vi "Sequencer.201806.vi"() -> ()   [LabVIEW 2014]
uses:
  Wave.ctl
  <vilib>/Analysis/NI_AALPro.lvlib
  <vilib>/gmath/NI_Gmath.lvlib
  <vilib>/gmath/statdist.llb/Poisson Random.vi
panel:
  out "Wave":T1 {"Phase (Pi)" min=-1.0 max=1.0 step=0.1 format="%.2f"; "Gap (us)" format="%.2f"; "Amplitude" format="%.2f"; "Duration (us)" format="%.2f"; "Frequency (MHz)" format="%.4f"}
  out "All Wave":T1 {"Phase (Pi)" min=-1.0 max=1.0 step=0.1 format="%.2f"; "Gap (us)" format="%.2f"; "Amplitude" format="%.2f"; "Duration (us)" format="%.2f"; "Frequency (MHz)" format="%.4f"}
  out "SegmentPositions":u32[](array[numeric])
  in  "All Wave (MHz, us, Pi)":string[][](table)=[["Frequency (MHz)", "Duration (us)", "Amplitude", "Phase (Pi)", "Gap (us)"], ["200.012", "100.000", "1.000", "0.000", "0.001"]]
  out "Item Function":refnum<vi>
  in  "Set":bool
  in  "Item":string(combo)="Time"
  out "SequenceNames":string[](array[string])
  in  "Parameter":u16(ring) items=["Frequency", "Amplitude", "Phase"]
  in  "Scan":bool
  out "Value":dbl=1.0 format="%.4f"
  in  "Step":dbl=1.0 format="%.4f"
  in  "End":dbl=1.0 format="%.3f"
  in  "Start":dbl=1.0 format="%.3f"
  out "Counts":u32[](array[numeric])
  out "CompiledSequence":string="#DopplerCooling\r\n0.9 10100000 00000000 00000000\r\n\r\n#Pump\r\n0.3 01000000 00000000 00000000\r\n\r\n#Pulsed\r\n0.2 00100000 00000000 00000000\r\n0.4 00000100 00000000 00000000\r\n0.2 00000000 10000000 00000000\r\n0.2 01000000 00000000 01000000\n"
  out "ChapterNames":string[](array[string])
  out "ChapterPositions":u32[](array[numeric])
  out "Durations Backup":dbl[](array[numeric])
  out "Durations":dbl[](array[numeric])
  in  "Period (ns)":dbl=5.0
  out "States":string[](array[string])
  in  "Sequencer":bool
  in  "Edit":enum32{"Sequence", "Wave"}(tab)
  in  "Sequence":string
  in  "Chapter (us)":string
  in  "Sequence File":path=path "D:/Data/Sequence/Cooling.seq"
  in  "Repeats":u32=100
  in  "Compile":bool
  in  "Send":bool
  in  "Port":refnum<visa-resource-name>="COM5"
  in  "Trigger":bool
  in  "Save":bool
  in  "Wave (MHz, us, Pi)":string[][](table)
  in  "Wave File":path=path "D:/Data/Wave/Test.csv"
  in  "Save":bool
  in  "Load":bool
  in  "Segment":u16(ring) items=["0"]
  in  "Index":u16(ring) items=["0", "1", "All"]
  in  "Channel":u16(ring) items=["0"]
  in  "Mode":u16(ring) items=["0"]
  out "Clock":string
  in  "Detect":enum32{"PMT", "AWG", "CCD"}(tab)
  in  "4":bool
  in  "3":bool
  in  "2":bool
  in  "1":bool=TRUE
  in  "Count or State":i16(ring) items=["Count", "State"]
  in  "Fit":bool
  out "Peak":u32
  out "?":cluster{"Axis":dbl[], "Histogram":i32[]}(graph)
  in  "Data Chapter":i16(ring) items=["All", "Detection[2]"]
  out "Average Counts or States":dbl(graph)
  out "data file":string
  out "History":dbl[](array[numeric])
  in  "Sweep":bool
  in  "Clear":bool
  in  "Data":bool
  in  "Threshold":dbl=1.0
  out "Graph":waveform(dbl)(graph)
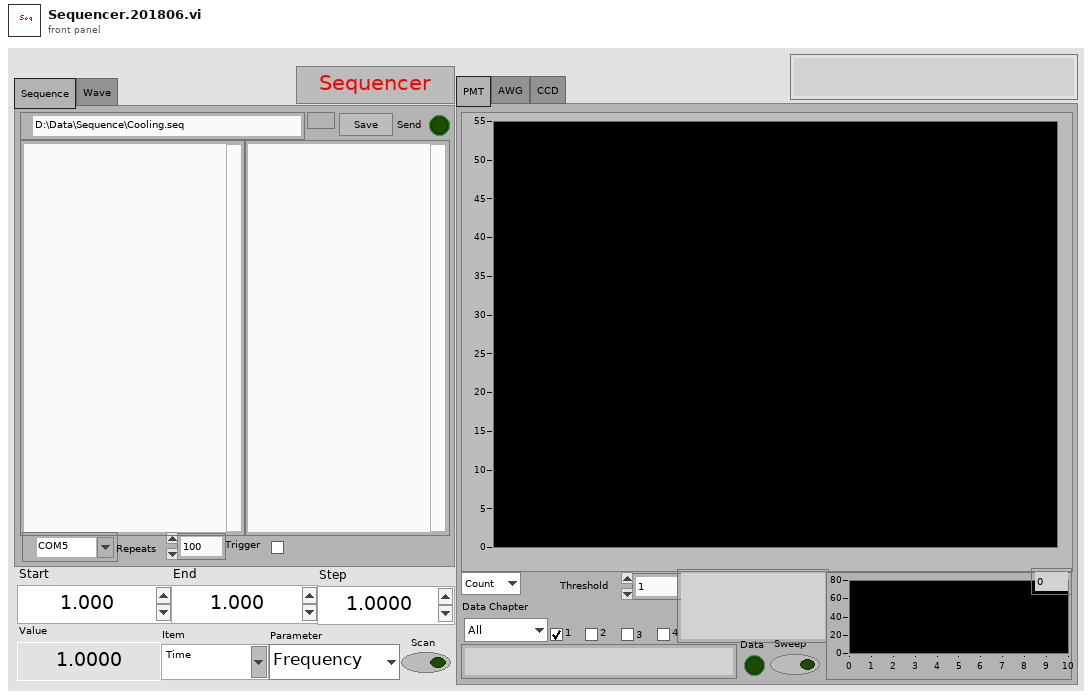
[diagram p1: front panel]
types:
  T1 = typedef "Wave.ctl" = cluster{"Frequency (MHz)":dbl, "Duration (us)":dbl, "Amplitude":dbl, "Phase (Pi)":dbl, "Gap (us)":dbl, "Formula":string}[]
  T2 = cluster{"lower":dbl, "upper":dbl, "inclusion":enum32{"lower", "upper", "both", "neither"}}[]
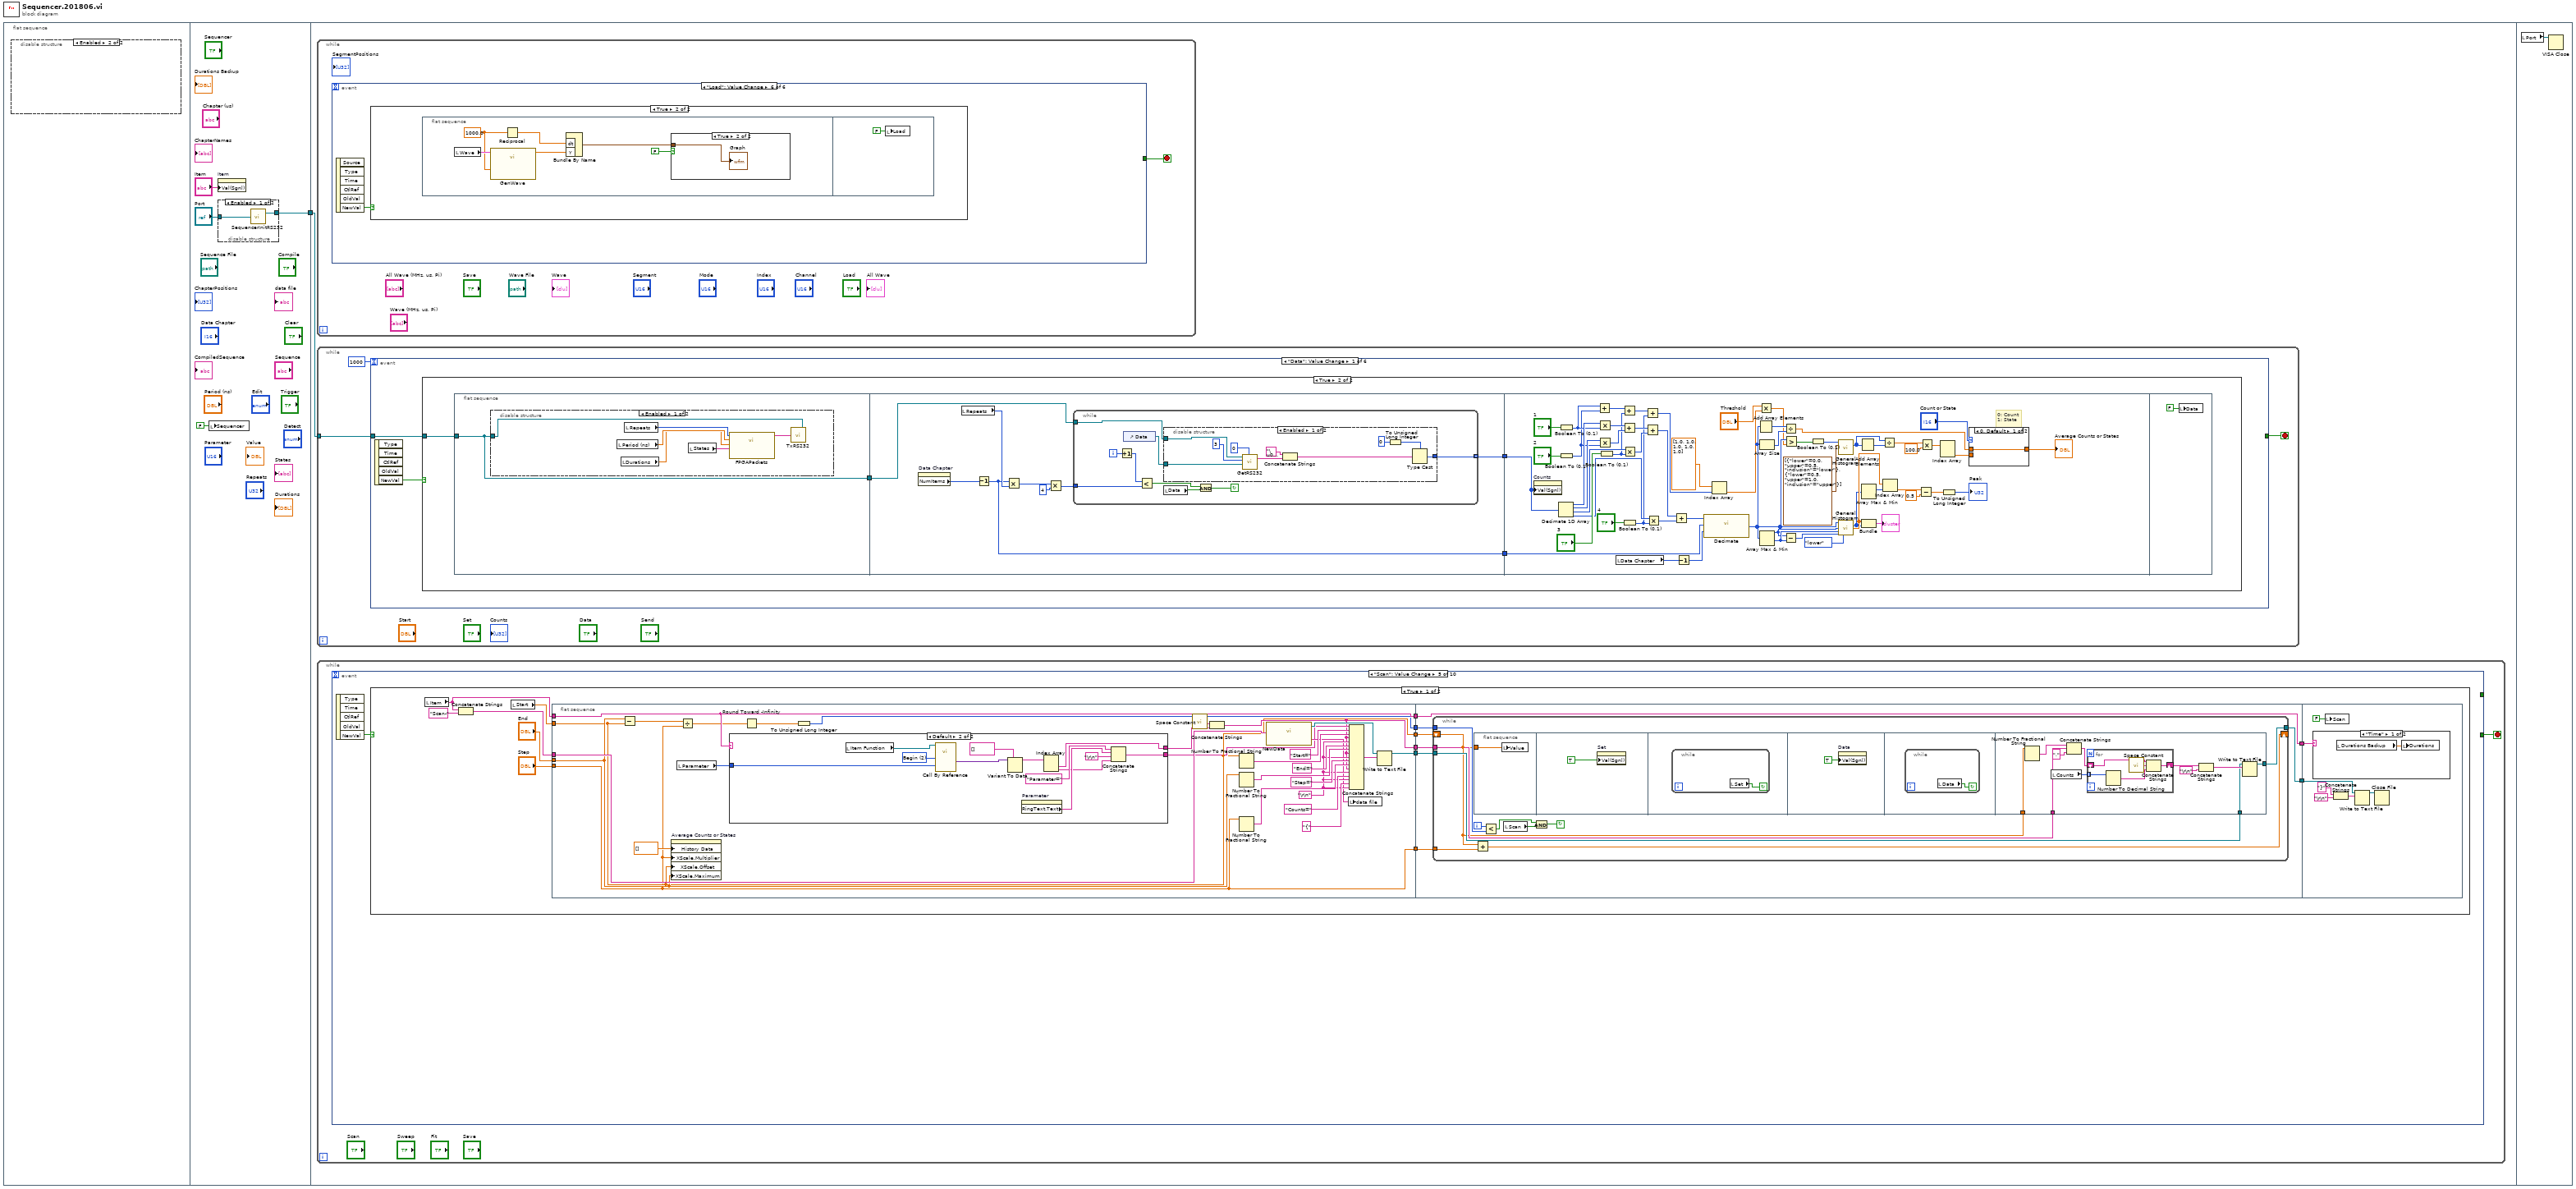
[diagram p0: block diagram]
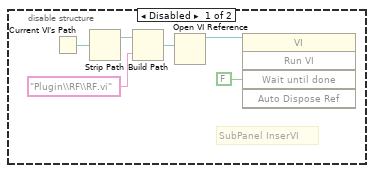
[diagram p2: hidden frame]
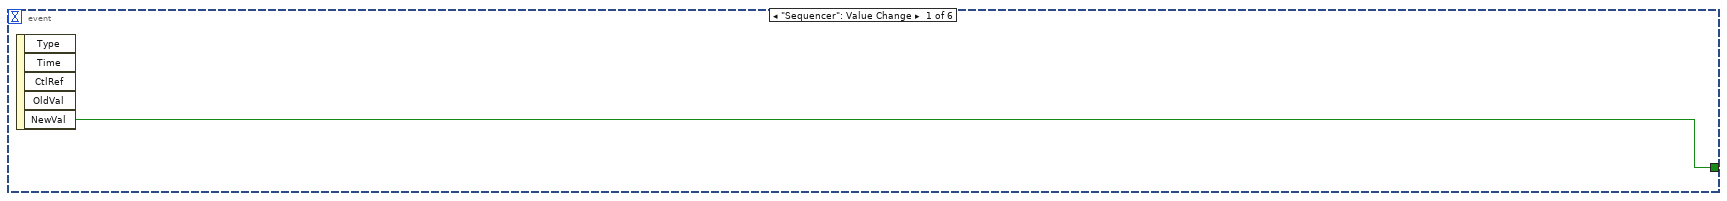
[diagram p4: hidden frame]
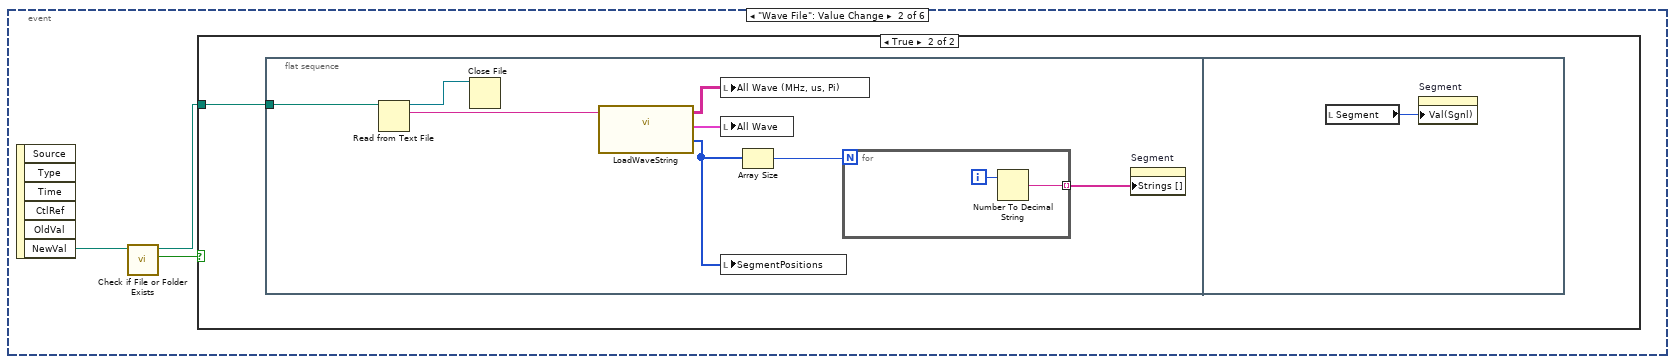
[diagram p5: hidden frame]
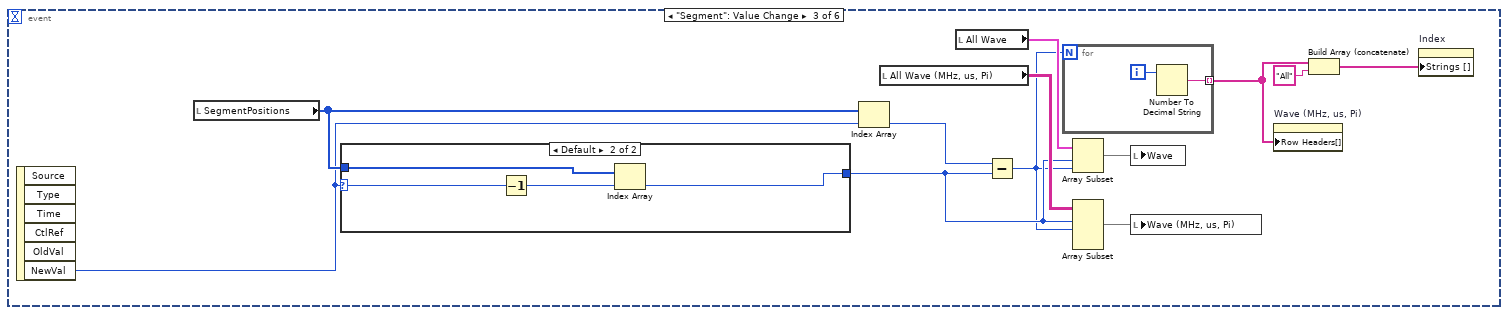
[diagram p7: hidden frame]
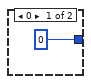
[diagram p8: hidden frame]
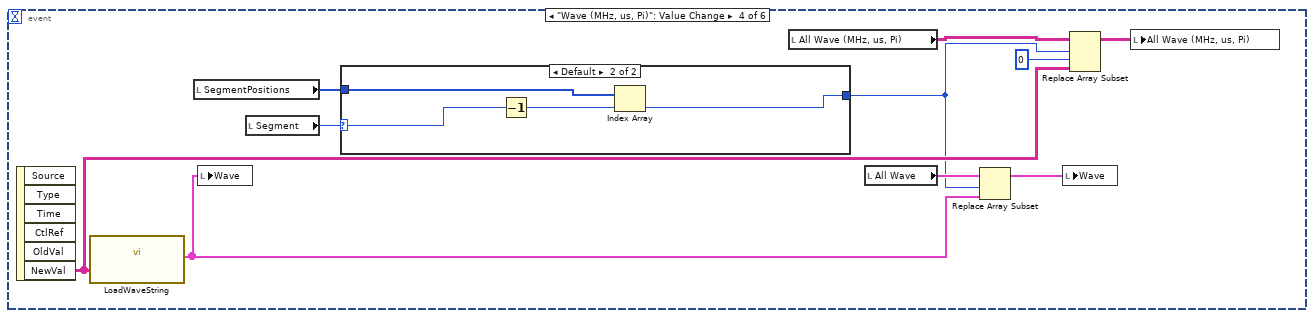
[diagram p9: hidden frame]
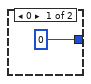
[diagram p10: hidden frame]
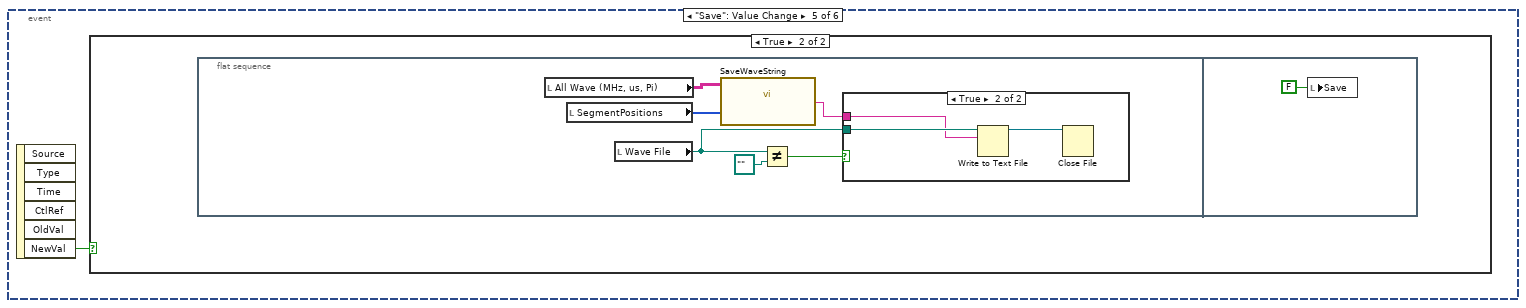
[diagram p11: hidden frame]
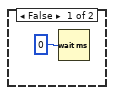
[diagram p16: hidden frame]
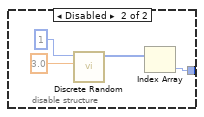
[diagram p18: hidden frame]
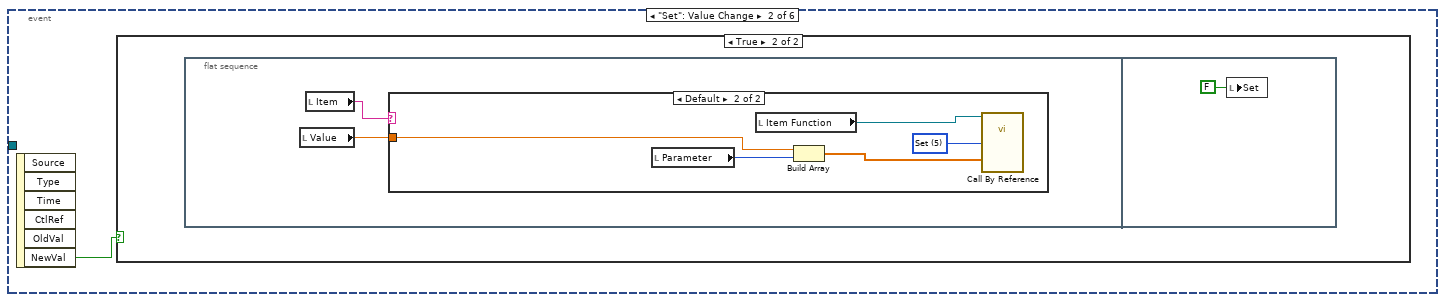
[diagram p20: hidden frame]
diagram:
  n1 = flat-sequence {
    tunnel: [w9] -> w1
    tunnel: w1 -> [w14]
    frame #0 {
      n2 = disable-structure shown="Enabled" {
        frame Disabled {
          # "SubPanel InserVI"
          n3 = Current VI's Path() -> (path=w4:path)
          n4 = Strip Path(path=w4) -> (stripped path=w6:path)  [unwired: 1 out]
          n5 = Build Path(base path=w6, name or relative path="Plugin\\RF\\RF.vi") -> (appended path=w5:path)
          n6 = Open VI Reference(vi path=w5) -> (vi reference=w3:refnum<vi>)  [unwired: 5 in, 1 out]
          n7 = invoke class="VI" method="Run VI"(reference=w3, "Wait until done"=FALSE ("Wait Until Done")) -> ()  [unwired: 3 in, 5 out]
        }
        frame Enabled {
        }
      }
    }
    frame #1 {
      n8 = local write "Sequencer"(FALSE ("Sequencer")) -> ()
      n9 = property on="Item" class="CmbBox"("Val(Sgnl)"="Item") -> ()  [unwired: 2 in, 2 out]
      n10 = disable-structure shown="Enabled" {
        disable-tunnel: "Port" -> [w13 _]
        disable-tunnel: [w12 _] -> w9
        frame Enabled {
          n11 = call "SequencerInitRS232.vi"("VISA resource name"=w13) -> ("reference out"=w12:refnum<visa-resource-name>)  [unwired: 1 out]
        }
        frame Disabled {
        }
      }
    }
    frame #2 {
      n12 = while {
        stop <- w15 stop-if-true
        n13 = event shown="[5] \"Load\": Value Change" {
          selector: _ -> [_ _ _ _ _ _]
          dyn-events: _ -> [_ _ _ _ _ _]
          timeout: _ -> [_ _ _ _ _ _]
          tunnel: [w16 _ _ _ _ _] -> w15
          event "Sequencer": Value Change {
            n14 = event-data() -> ("NewVal"=w16:bool)  [unwired: 1 in, 4 out]
          }
          event "Wave File": Value Change {
            n15 = event-data() -> ("NewVal"=w19:path)  [unwired: 1 in, 5 out]
            n16 = call <vilib>:"Check if File or Folder Exists.vi"("path"=w19) -> ("file or folder exists?"=w18:bool, "dup path"=w17:path)  [unwired: 8 in, 1 out]
            n17 = case shown="True" w18 {
              tunnel: w17 -> [_ w20]
              frame False {
              }
              frame True {
                n18 = flat-sequence {
                  tunnel: w20 -> [w27]
                  frame #0 {
                    n19 = Read from Text File(file (use dialog)=w27) -> (refnum out=w28:refnum<file>, text=w21:string)  [unwired: 3 in, 2 out]
                    n20 = Close File(refnum=w28) -> ()  [unwired: 1 in, 2 out]
                    n21 = call "LoadWaveString.vi"("Wave String"=w21) -> ("All Wave (MHz,us)"=w26:string[][], "All Wave"=w25:T1, "SegmentPositions"=w22:i32[])  [unwired: 1 in]
                    n22 = local write "All Wave (MHz, us, Pi)"(w26) -> ()
                    n23 = local write "All Wave"(w25) -> ()
                    n24 = local write "SegmentPositions"(w22) -> ()
                    n25 = Array Size(array=w22) -> (size(s)=w23:i32)
                    n26 = for {
                      N: w23 -> [_]
                      tunnel: [w29] -> w24 mode=indexing
                      i -> [w30]
                      n27 = Number To Decimal String(number=w30) -> (decimal integer string=w29:string)  [unwired: 1 in]
                    }
                    n28 = property on="Segment" class="Ring (strict)"("Strings []"=w24) -> ()  [unwired: 2 in, 2 out]
                  }
                  frame #1 {
                    n29 = local read "Segment"() -> (w31:u16)
                    n30 = property on="Segment" class="Ring (strict)"("Val(Sgnl)"=w31) -> ()  [unwired: 2 in, 2 out]
                  }
                }
              }
            }
          }
          event "Segment": Value Change {
            n31 = event-data() -> ("NewVal"=w33:u16)  [unwired: 1 in, 5 out]
            n32 = local read "SegmentPositions"() -> (w43:u32[])
            n33 = case shown="Default" w33 {
              selector: w33 -> [_ w45]
              tunnel: [0 w46] -> w38
              tunnel: w43 -> [_ w47]
              frame 0 {
              }
              frame Default {
                n34 = Decrement(x=w45) -> (x-1=w48:u16)
                n35 = Index Array(array=w47, index=w48) -> (element=w46:u32)
              }
            }
            n36 = Index Array(array=w43, index=w33) -> (element=w42:u32)
            n37 = local read "All Wave (MHz, us, Pi)"() -> (w41:string[][])
            n38 = local read "All Wave"() -> (w39:T1)
            n39 = Subtract(x=w42, y=w38) -> (x-y=w36:u32)
            n40 = for {
              N: w36 -> [_]
              tunnel: [w49] -> w32 mode=indexing
              i -> [w50]
              n41 = Number To Decimal String(number=w50) -> (decimal integer string=w49:string)  [unwired: 1 in]
            }
            n42 = Array Subset(array=w39, index=w38, length=w36) -> (w37:T1)
            n43 = Array Subset(array=w41, index (row)=w38, length (row)=w36) -> (w40:string[][])  [unwired: 2 in]
            n44 = local write "Wave"(w37) -> ()
            n45 = local write "Wave (MHz, us, Pi)"(w40) -> ()
            n46 = property on="Wave (MHz, us, Pi)" class="Tbl (strict)"("Row Headers[]"=w32) -> ()  [unwired: 2 in, 2 out]
            n47 = Build Array (concatenate)(w32, "All") -> (w35:string[])
            n48 = property on="Index" class="Ring (strict)"("Strings []"=w35) -> ()  [unwired: 2 in, 2 out]
          }
          event "Wave (MHz, us, Pi)": Value Change {
            n49 = event-data() -> ("NewVal"=w56:string[][])  [unwired: 1 in, 5 out]
            n50 = call "LoadWaveString.vi"("Wave (MHz,us,Pi)"=w56) -> ("All Wave"=w51:T1)  [unwired: 1 in, 2 out]
            n51 = local read "SegmentPositions"() -> (w60:u32[])
            n52 = local write "Wave"(w51) -> ()
            n53 = local read "Segment"() -> (w59:u16)
            n54 = case shown="Default" w59 {
              selector: w59 -> [_ w62]
              tunnel: [0 w63] -> w53
              tunnel: w60 -> [_ w64]
              frame 0 {
              }
              frame Default {
                n55 = Decrement(x=w62) -> (x-1=w65:u16)
                n56 = Index Array(array=w64, index=w65) -> (element=w63:u32)
              }
            }
            n57 = local read "All Wave (MHz, us, Pi)"() -> (w58:string[][])
            n58 = local read "All Wave"() -> (w54:T1)
            n59 = Replace Array Subset(array=w54, new element=w51, index=w53) -> (w52:T1)
            n60 = local write "Wave"(w52) -> ()
            n61 = Replace Array Subset(array=w58, new element=w56, index (row)=w53, index (col)=0 ("disabled index (col)")) -> (w55:string[][])
            n62 = local write "All Wave (MHz, us, Pi)"(w55) -> ()
          }
          event "Save": Value Change {
            n63 = event-data() -> ("NewVal"=w66:bool)  [unwired: 1 in, 5 out]
            n64 = case shown="True" w66 {
              frame False {
              }
              frame True {
                n65 = flat-sequence {
                  frame #0 {
                    n66 = local read "All Wave (MHz, us, Pi)"() -> (w70:string[][])
                    n67 = local read "SegmentPositions"() -> (w71:u32[])
                    n68 = local read "Wave File"() -> (w68:path)
                    n69 = call "SaveWaveString.vi"("SegmentPositions"=w71, "All Wave (MHz,us)"=w70) -> ("String"=w67:string)
                    n70 = Not Equal?(x=w68, y=path "") -> (x != y?=w69:bool)
                    n71 = case shown="True" w69 {
                      tunnel: w68 -> [_ w75]
                      tunnel: w67 -> [_ w74]
                      frame False {
                      }
                      frame True {
                        n72 = Write to Text File(file (use dialog)=w75, text=w74) -> (refnum out=w73:refnum<file>)  [unwired: 2 in, 2 out]
                        n73 = Close File(refnum=w73) -> ()  [unwired: 1 in, 2 out]
                      }
                    }
                  }
                  frame #1 {
                    n74 = local write "Save"(FALSE ("Save")) -> ()
                  }
                }
              }
            }
          }
          event "Load": Value Change {
            n75 = event-data() -> ("NewVal"=w77:bool)  [unwired: 1 in, 5 out]
            n76 = case shown="True" w77 {
              frame False {
              }
              frame True {
                n77 = flat-sequence {
                  frame #0 {
                    w80 = 1000.0 ("x")
                    n78 = local read "Wave"() -> (w83:T1)
                    n79 = call "GenWave.vi"("Sampling Rate (MHz)"=w80, "Wave"=w83) -> ("Output"=w79:dbl[])  [unwired: 4 in, 1 out]
                    n80 = Reciprocal(x=w80) -> (1/x=w81:dbl)
                    n81 = Bundle By Name("dt"=w81, "Y"=w79) -> (w82:waveform(dbl))  [unwired: 1 in]
                    n82 = case shown="True" FALSE ("Show") {
                      tunnel: w82 -> [_ w84]
                      frame False {
                      }
                      frame True {
                        "Graph" <- w84
                      }
                    }
                  }
                  frame #1 {
                    n83 = local write "Load"(FALSE ("Load")) -> ()
                  }
                }
              }
            }
          }
        }
      }
      n84 = while {
        tunnel: w14 -> [w88]
        stop <- w87 stop-if-true
        n85 = event shown="[0] \"Data\": Value Change" {
          selector: _ -> [_ _ _ _ _ _]
          dyn-events: _ -> [_ _ _ _ _ _]
          timeout: u32 1000 ("milliseconds to wait") -> [_ _ _ _ _ _]
          tunnel: w88 -> [w90 _ _ _ _ w214]
          tunnel: [_ _ _ _ w213 _] -> w87
          event "Data": Value Change {
            n86 = event-data() -> ("NewVal"=w89:bool)  [unwired: 1 in, 4 out]
            n87 = case shown="True" w89 {
              tunnel: w90 -> [_ w95]
              frame False {
                n88 = Wait (ms)(milliseconds to wait=u32 0) -> ()  [unwired: 1 out]
              }
              frame True {
                n89 = flat-sequence {
                  tunnel: w95 -> [w96]
                  tunnel: [w96] -> w92
                  tunnel: [w108] -> w94
                  tunnel: [w106] -> w93
                  tunnel: w92 -> [w110]
                  tunnel: w94 -> [w160]
                  tunnel: w93 -> [w165]
                  frame #0 {
                    n90 = disable-structure shown="Enabled" {
                      disable-tunnel: w96 -> [w101 _]
                      frame Enabled {
                        n91 = local read "Period (ns)"() -> (w99:dbl)
                        n92 = local read "Durations"() -> (w98:dbl[])
                        n93 = local read "Repeats"() -> (w100:u32)
                        n94 = local read "States"() -> (w97:string[])
                        n95 = call "FPGAPackets.vi"("Repeats"=w100, "Period (ns)"=w99, "Durations"=w98, "States"=w97) -> ("Packets"=w102:string)  [unwired: 1 in, 1 out]
                        n96 = call "TxRS232.vi"("VISA resource name"=w101, "Data"=w102) -> ()
                      }
                      frame Disabled {
                      }
                    }
                  }
                  frame #1 {
                    n97 = property on="Data Chapter" class="Ring (strict)"() -> ("NumItems"=w109:u32)  [unwired: 2 in, 2 out]
                    n98 = local read "Repeats"() -> (w107:u32)
                    n99 = Decrement(x=w109) -> (x-1=w106:u32)
                    n100 = Multiply(x=w106, y=w107) -> (x*y=w105:u32)
                    n101 = Multiply(x=w105, y=u32 4) -> (x*y=w104:u32)
                    n102 = while {
                      tunnel: w110 -> [w115]
                      tunnel: [w116] -> w108 mode=indexing
                      tunnel: w104 -> [w113]
                      i -> [w112]
                      stop <- w118 continue-if-true
                      n103 = Increment(x=w112) -> (x+1=w111:i32)
                      n104 = control-ref of="Data"() -> (w114:refnum<vi>)
                      n105 = Less?(x=w111, y=w113) -> (x < y?=w117:bool)
                      n106 = disable-structure shown="Enabled" {
                        disable-tunnel: [w125 w130] -> w116
                        disable-tunnel: w115 -> [w124 _]
                        disable-tunnel: w114 -> [w121 _]
                        frame Enabled {
                          n107 = call "GetRS232.vi"("VISA resource name"=w124, "Bytes To Read"=3, "Control"=w121, "Limit"=0) -> ("Data"=w122:string)  [unwired: 1 in, 1 out]
                          n108 = Concatenate Strings("\u0000" ("string"), w122) -> (w126:string)
                          n109 = To Unsigned Long Integer(number=u32 0) -> (unsigned 32bit integer=w129:u32)
                          n110 = Type Cast(type=w129, x=w126) -> (*(type *) &x=w125:u32)
                        }
                        frame Disabled {
                          n111 = call-poly <vilib>:"Discrete Random.vi"("lambda"=3.0, "samples"=1) -> ("Poisson random data"=w131:i32[])  [unwired: 8 in, 1 out]
                          n112 = Index Array(array=w131) -> (element=w130:i32)  [unwired: 1 in]
                        }
                      }
                      n113 = local read "Data"() -> (w119:bool)
                      n114 = And(x=w117, y=w119) -> (x .and. y?=w118:bool)
                    }
                  }
                  frame #2 {
                    # "0: Count\n1: State"
                    n115 = property on="Counts" class="Arr (strict)"("Val(Sgnl)"=w160) -> ()  [unwired: 2 in, 2 out]
                    n116 = Boolean To (0,1)(Boolean="1") -> (0, 1=w144:i16)
                    n117 = Boolean To (0,1)(Boolean="2") -> (0, 1=w143:i16)
                    n118 = Decimate 1D Array(w160) -> (w159:u32[], w156:u32[], w152:u32[], w149:u32[])
                    n119 = Add(x=w144, y=w143) -> (x+y=w142:i16)
                    n120 = Multiply(x=w159, y=w144) -> (x*y=w145:u32[])
                    n121 = Multiply(x=w156, y=w143) -> (x*y=w155:u32[])
                    n122 = Boolean To (0,1)(Boolean="3") -> (0, 1=w141:i16)
                    n123 = local read "Data Chapter"() -> (w163:i16)
                    n124 = Add(x=w142, y=w141) -> (x+y=w140:i16)
                    n125 = Add(x=w145, y=w155) -> (x+y=w150:u32[])
                    n126 = Multiply(x=w152, y=w141) -> (x*y=w151:u32[])
                    n127 = Boolean To (0,1)(Boolean="4") -> (0, 1=w139:i16)
                    n128 = Add(x=w140, y=w139) -> (x+y=w134:i16)
                    n129 = Add(x=w150, y=w151) -> (x+y=w147:u32[])
                    n130 = Multiply(x=w149, y=w139) -> (x*y=w148:u32[])
                    n131 = Add(x=w147, y=w148) -> (x+y=w146:u32[])
                    n132 = Decrement(x=w163) -> (x-1=w162:i16)
                    n133 = call "Decimate.vi"("i"=w162, "n"=w165, "Input Array"=w146) -> ("Decimated Array"=w186:u32[])
                    n134 = Index Array(array=dbl[] [1.0, 1.0, 1.0, 1.0, 1.0], index=w134) -> (element=w136:dbl)
                    n135 = Multiply(x="Threshold", y=w136) -> (x*y=w135:dbl)
                    n136 = Add Array Elements(numeric array=w186) -> (sum=w185:u32)
                    n137 = Array Size(array=w186) -> (size(s)=w184:i32)
                    n138 = Array Max & Min(array=w186) -> (max value=w166:u32, min value=w175:u32)  [unwired: 2 out]
                    n139 = Divide(x=w185, y=w184) -> (x/y=w188:dbl)
                    n140 = Subtract(x=w166, y=w175) -> (x-y=w174:u32)
                    n141 = Greater?(x=w186, y=w135) -> (0:w172:bool[])
                    n142 = Boolean To (0,1)(Boolean=w172) -> (0, 1=w171:i16[])
                    n143 = call <vilib>:"General Histogram.vi"("X"=w171, "Bins"=T2 [{"lower"=0.0, "upper"=0.5, "inclusion"=enum."lower"}, {"lower"=0.5, "upper"=1.0, "inclusion"=enum."upper"}]) -> ("Histogram"=w169:i32[])  [unwired: 9 in, 4 out]
                    n144 = call <vilib>:"General Histogram.vi"("X"=w186, "max"=w166, "min"=w175, "# bins"=w174, "inclusion"=enum32{"lower", "upper"}."lower") -> ("Histogram"=w176:i32[], "Axis"=w178:dbl[])  [unwired: 6 in, 3 out]
                    n145 = Add Array Elements(numeric array=w169) -> (sum=w170:i32)
                    n146 = Array Max & Min(array=w176) -> (max index (indices)=w177:i32)  [unwired: 3 out]
                    n147 = Bundle("Axis"=w178, "Histogram"=w176) -> (→"?":cluster{"Axis":dbl[], "Histogram":i32[]})  [unwired: 1 in]
                    n148 = Divide(x=w169, y=w170) -> (x/y=w167:dbl[])
                    n149 = Index Array(array=w178, index=w177) -> (element=w182:dbl)
                    n150 = Subtract(x=w182, y=0.5) -> (x-y=w181:dbl)
                    n151 = Multiply(x=w167, y=100.0) -> (x*y=w187:dbl[])
                    n152 = Index Array(array=w187) -> (element #2=w189:dbl)  [unwired: 2 in, 1 out]
                    n153 = To Unsigned Long Integer(number=w181) -> (unsigned 32bit integer=→"Peak":u32)
                    n154 = case shown="0, Default" "Count or State" {
                      tunnel: w188 -> [w191 _]
                      tunnel: [w191 w192] -> w190
                      tunnel: w189 -> [_ w192]
                      frame 0, Default {
                      }
                      frame 1 {
                      }
                    }
                    "Average Counts or States" <- w190
                  }
                  frame #3 {
                    n155 = local write "Data"(FALSE ("Acquisition")) -> ()
                  }
                }
              }
            }
          }
          event "Set": Value Change {
            n156 = event-data() -> ("NewVal"=w194:bool)  [unwired: 1 in, 5 out]
            n157 = case shown="True" w194 {
              frame False {
              }
              frame True {
                n158 = flat-sequence {
                  frame #0 {
                    n159 = local read "Value"() -> (w195:dbl)
                    n160 = local read "Item"() -> (w196:string)
                    n161 = case shown="Default" w196 {
                      tunnel: w195 -> [w197 w203]
                      frame "Time" {
                        n162 = local read "Parameter"() -> (w200:u16)
                        n163 = local read "Durations"() -> (w198:dbl[])
                        n164 = Replace Array Subset(array=w198, new element=w197, index=w200) -> (w199:dbl[])
                        n165 = local write "Durations"(w199) -> ()
                      }
                      frame Default {
                        w204 = u32 5 items=["Open", "Close", "Begin", "End", "Get", "Set"] ("Mode")
                        n166 = local read "Parameter"() -> (w202:u16)
                        n167 = local read "Item Function"() -> (w205:refnum<vi>)
                        n168 = Build Array(w203, w202) -> (w201:dbl[])
                        n169 = call-by-ref "?"(reference=w205, "In"=w201, "Mode"=w204) -> ()  [unwired: 1 in, 3 out]
                      }
                    }
                  }
                  frame #1 {
                    n170 = local write "Set"(FALSE ("Ready")) -> ()
                  }
                }
              }
            }
          }
          event Timeout {
            n171 = event-data() -> ()  [unwired: 1 in, 3 out]
            n172 = Get Date/Time In Seconds() -> (seconds since 1Jan1904=w207:timestamp)
            n173 = Format Date/Time String(time format string (%c)="%Y/%m/%d %H:%M:%S", seconds (now)=w207) -> (date/time string=→"Clock":string)  [unwired: 1 in]
          }
          event "Start": Value Change {
            n174 = event-data() -> ("NewVal"=w210:dbl)  [unwired: 1 in, 5 out]
            n175 = flat-sequence {
              tunnel: w210 -> [w211]
              frame #0 {
                n176 = local write "Value"(w211) -> ()
              }
              frame #1 {
                n177 = property on="Set" class="Bool (strict)"("Val(Sgnl)"=TRUE ("Value (Signaling)")) -> ()  [unwired: 2 in, 2 out]
              }
            }
          }
          event "Sequencer": Value Change {
            n178 = event-data() -> ("NewVal"=w213:bool)  [unwired: 1 in, 4 out]
          }
          event "Send": Value Change {
            n179 = event-data() -> ("NewVal"=w215:bool)  [unwired: 1 in, 4 out]
            n180 = case shown="True" w215 {
              tunnel: w214 -> [_ w216]
              frame False {
              }
              frame True {
                n181 = flat-sequence {
                  tunnel: w216 -> [w217]
                  frame #0 {
                    n182 = local read "Period (ns)"() -> (w221:dbl)
                    n183 = local read "Durations"() -> (w219:dbl[])
                    n184 = local read "Repeats"() -> (w220:u32)
                    n185 = local read "States"() -> (w222:string[])
                    n186 = call "FPGAPackets.vi"("Repeats"=w220, "Period (ns)"=w221, "Durations"=w219, "States"=w222) -> ("Packets"=w218:string)  [unwired: 1 in, 1 out]
                    n187 = call "TxRS232.vi"("VISA resource name"=w217, "Data"=w218) -> ()
                  }
                  frame #1 {
                    n188 = local write "Send"(FALSE ("Send")) -> ()
                  }
                }
              }
            }
          }
        }
      }
      n189 = while {
        stop <- w224 stop-if-true
        n190 = event shown="[4] \"Scan\": Value Change" {
          selector: _ -> [_ _ _ _ _ _ _ _ _ _]
          dyn-events: _ -> [_ _ _ _ _ _ _ _ _ _]
          timeout: _ -> [_ _ _ _ _ _ _ _ _ _]
          tunnel: [_ _ _ _ _ _ _ _ _ w530] -> _
          tunnel: [_ _ _ _ _ _ _ _ _ w530] -> w224
          event "Compile": Value Change {
            n191 = event-data() -> ("NewVal"=w225:bool)  [unwired: 1 in, 4 out]
            n192 = case shown="True" w225 {
              frame False {
              }
              frame True {
                n193 = flat-sequence {
                  frame #0 {
                    n194 = disable-structure shown="Disabled" {
                      frame Disabled {
                        n195 = local read "Chapter (us)"() -> (w242:string)
                        n196 = local read "Sequence"() -> (w241:string)
                        n197 = call "CompileSequence.vi"("Sequence"=w241, "Chapter"=w242) -> ("Compiled Sequence"=w240:string)
                        n198 = local write "CompiledSequence"(w240) -> ()
                      }
                      frame Enabled {
                      }
                    }
                    n199 = local read "CompiledSequence"() -> (w228:string)
                    n200 = call "LoadCompiledString.vi"("Compiled String"=w228) -> ("Durations"=w237:dbl[], "States"=w236:string[], "ChapterNames"=w229:string[], "ChapterPositions"=w230:u32[])
                    n201 = local write "States"(w236) -> ()
                    n202 = local write "ChapterPositions"(w230) -> ()
                    n203 = for {
                      tunnel: w230 -> [w243] mode=indexing
                      tunnel: w229 -> [w244] mode=indexing
                      shift-right: [w243] -> _
                      shift-left: u32 0 ("initial scan location") -> [w250]
                      shift-right: [w245] -> w226
                      shift-left: string[] [] -> [w246]
                      n204 = Subtract(x=w243, y=w250) -> (x-y=w247:u32)
                      n205 = Greater?(x=w247, y=u32 1) -> (0:w249:bool)
                      n206 = case shown="True" w249 {
                        tunnel: w244 -> [w252 w258]
                        tunnel: w247 -> [_ w257]
                        tunnel: w246 -> [w253 w256]
                        tunnel: [w251 w254] -> w245
                        frame False {
                          n207 = Build Array (concatenate)(w253, w252) -> (w251:string[])
                        }
                        frame True {
                          n208 = for {
                            N: w257 -> [_]
                            tunnel: w258 -> [w263]
                            tunnel: [w262] -> w255 mode=indexing
                            i -> [w264]
                            n209 = Number To Octal String(2:w264) -> (0:w261:string)  [unwired: 1 in]
                            n210 = Concatenate Strings(w263, "[" ("string"), w261, "]" ("string")) -> (w262:string)
                          }
                          n211 = Build Array (concatenate)(w256, w255) -> (w254:string[])
                        }
                      }
                    }
                    "SequenceNames" <- w226
                    n212 = local write "Durations"(w237) -> ()
                    n213 = local write "ChapterNames"(w229) -> ()
                    n214 = for {
                      N -> [w276]
                      tunnel: w236 -> [w285] mode=indexing
                      shift-right: [w273] -> _
                      shift-left: "0" -> [w283]
                      tunnel: w229 -> [w279]
                      shift-right: [w268] -> w232
                      shift-left: string[] ["All"] -> [w267]
                      tunnel: w230 -> [w266]
                      i -> [w277]
                      n215 = Equal?(x=w283, y="1") -> (x = y?=w281:bool)
                      n216 = String Subset(string=w285, offset (0)=27, length (rest)=1 ("length (rest)")) -> (substring=w273:string)
                      n217 = Decrement(x=w276) -> (x-1=w275:i32)
                      n218 = Equal?(x=w277, y=w275) -> (x = y?=w272:bool)
                      n219 = Equal?(x=w273, y="1") -> (x = y?=w271:bool)
                      n220 = Equal?(x=w273, y="0") -> (x = y?=w278:bool)
                      n221 = And(x=w272, y=w271) -> (x .and. y?=w270:bool)
                      n222 = And(x=w281, y=w278) -> (x .and. y?=w269:bool)
                      n223 = case shown="True" w270 {
                        tunnel: w279 -> [w291 w331]
                        tunnel: w267 -> [w290 w333]
                        tunnel: w277 -> [w289 _]
                        tunnel: w269 -> [w288 _]
                        tunnel: [w287 w332] -> w268
                        tunnel: w266 -> [w286 w325]
                        frame False {
                          n224 = case shown="True" w288 {
                            tunnel: w289 -> [_ w303]
                            tunnel: w291 -> [_ w304]
                            tunnel: w290 -> [w292 w306]
                            tunnel: [w292 w307] -> w287
                            tunnel: w286 -> [_ w300]
                            frame False {
                            }
                            frame True {
                              n225 = Threshold 1D Array(2:w303, 3:w300) -> (0:w305:dbl)  [unwired: 1 in]
                              n226 = Round Toward +Infinity(x=w305) -> (ceil(x): smallest int >= x=w298:dbl)
                              n227 = Index Array(array=w300, index=w298) -> (element=w297:u32)
                              n228 = Index Array(array=w304, index=w298) -> (element=w301:string)
                              n229 = Decrement(x=w298) -> (x-1=w299:dbl)
                              n230 = Index Array(array=w300, index=w299) -> (element=w293:u32)
                              n231 = Subtract(x=w297, y=w293) -> (x-y=w296:u32)
                              n232 = Greater?(x=w296, y=u32 1) -> (0:w294:bool)
                              n233 = case shown="True" w294 {
                                tunnel: w303 -> [_ w317]
                                tunnel: [w308 w311] -> w302
                                tunnel: w301 -> [w308 w310]
                                tunnel: w293 -> [_ w309]
                                frame False {
                                }
                                frame True {
                                n234 = Subtract(x=w317, y=w309) -> (x-y=w316:u32)
                                n235 = Decrement(x=w316) -> (x-1=w315:u32)
                                n236 = Number To Decimal String(number=w315) -> (decimal integer string=w312:string)  [unwired: 1 in]
                                n237 = Concatenate Strings(w310, "[" ("element"), w312, "]" ("element")) -> (w311:string)
                                }
                              }
                              n238 = Build Array (concatenate)(w306, w302) -> (w307:string[])
                            }
                          }
                        }
                        frame True {
                          n239 = Array Size(array=w331) -> (size(s)=w330:i32)
                          n240 = Array Size(array=w325) -> (size(s)=w328:i32)
                          n241 = Decrement(x=w330) -> (x-1=w329:i32)
                          n242 = Decrement(x=w328) -> (x-1=w327:i32)
                          n243 = Index Array(array=w325, index=w327) -> (element=w324:u32)
                          n244 = Index Array(array=w331, index=w329) -> (element=w320:string)
                          n245 = Decrement(x=w327) -> (x-1=w326:i32)
                          n246 = Index Array(array=w325, index=w326) -> (element=w323:u32)
                          n247 = Subtract(x=w324, y=w323) -> (x-y=w318:u32)
                          n248 = Greater?(x=w318, y=u32 1) -> (0:w321:bool)
                          n249 = case shown="True" w321 {
                            tunnel: w320 -> [w334 w341]
                            tunnel: [w334 w335] -> w319
                            tunnel: w318 -> [_ w338]
                            frame False {
                            }
                            frame True {
                              n250 = Decrement(x=w338) -> (x-1=w337:u32)
                              n251 = Number To Octal String(2:w337) -> (0:w336:string)  [unwired: 1 in]
                              n252 = Concatenate Strings(w341, "[" ("string"), w336, "]" ("string")) -> (w335:string)
                            }
                          }
                          n253 = Build Array (concatenate)(w333, w319) -> (w332:string[])
                        }
                      }
                    }
                    n254 = local read "Item"() -> (w227:string)
                    n255 = case shown="\"Time\"" w227 {
                      tunnel: w226 -> [w239 _]
                      frame "Time" {
                        n256 = property on="Parameter" class="Ring (strict)"("Strings []"=w239) -> ()  [unwired: 2 in, 2 out]
                        n257 = local read "Parameter"() -> (w238:u16)
                        n258 = property on="Parameter" class="Ring (strict)"("Val(Sgnl)"=w238) -> ()  [unwired: 2 in, 2 out]
                      }
                      frame Default {
                      }
                    }
                    n259 = property on="Data Chapter" class="Ring (strict)"("Strings []"=w232) -> ()  [unwired: 2 in, 2 out]
                  }
                  frame #1 {
                    n260 = local write "Compile"(FALSE ("Compile")) -> ()
                  }
                }
              }
            }
          }
          event "Item": Value Change {
            n261 = event-data() -> ("NewVal"=w344:string)  [unwired: 1 in, 5 out]
            n262 = flat-sequence {
              tunnel: w344 -> [w348]
              tunnel: [w348] -> w343
              tunnel: w343 -> [w350]
              frame #0 {
                w347 = u32 1 items=["Open", "Close", "Begin", "End", "Get", "Set"] ("Mode")
                n263 = local read "Item Function"() -> (w346:refnum<vi>)
                n264 = call-by-ref "?"(reference=w346, "Mode"=w347) -> (error out=w345:errorcluster)  [unwired: 2 in, 2 out]
                n265 = call <vilib>:"Clear Errors.vi"("error in (no error)"=w345) -> ()  [unwired: 5 in, 2 out]
              }
              frame #1 {
                n266 = case shown="Default" w350 {
                  selector: w350 -> [w358 _]
                  tunnel: [w351 w363] -> w349
                  frame Default {
                    w354 = u32 0 items=["Open", "Close", "Begin", "End", "Get", "Set"] ("Mode")
                    n267 = Concatenate Strings(w358, ".vi" ("string")) -> (w356:string)
                    n268 = Current VI's Path() -> (path=w360:path)
                    n269 = Strip Path(path=w360) -> (stripped path=w359:path)  [unwired: 1 out]
                    n270 = Build Path(base path=w359, name or relative path=w356) -> (appended path=w361:path)
                    n271 = Open VI Reference(type specifier VI Refnum (for type only)=refnum<vi> refnum, vi path=w361) -> (vi reference=w355:refnum<vi>)  [unwired: 4 in, 1 out]
                    "Item Function" <- w355
                    n272 = call-by-ref "?"(reference=w355, "Mode"=w354) -> ("Out"=w353:variant)  [unwired: 2 in, 2 out]
                    n273 = Variant To Data(type=string[] [] ("Strings []"), Variant=w353) -> (data=w351:string[])  [unwired: 1 in, 1 out]
                  }
                  frame "Time" {
                    n274 = local read "SequenceNames"() -> (w363:string[])
                  }
                }
                n275 = property on="Parameter" class="Ring (strict)"("Strings []"=w349) -> ()  [unwired: 2 in, 2 out]
              }
              frame #2 {
                n276 = local read "Parameter"() -> (w364:u16)
                n277 = property on="Parameter" class="Ring (strict)"("Val(Sgnl)"=w364) -> ()  [unwired: 2 in, 2 out]
              }
            }
          }
          event "Parameter": Value Change {
            n278 = event-data() -> ("NewVal"=w365:u16)  [unwired: 1 in, 5 out]
            n279 = local read "Item"() -> (w367:string)
            n280 = case shown="\"Time\"" w367 {
              tunnel: [w369 w372] -> w366
              tunnel: w365 -> [w368 w371]
              frame "Time" {
                n281 = local read "Durations"() -> (w370:dbl[])
                n282 = Index Array(array=w370, index=w368) -> (element=w369:dbl)
              }
              frame Default {
                w375 = u32 4 items=["Open", "Close", "Begin", "End", "Get", "Set"] ("Mode")
                n283 = local read "Item Function"() -> (w376:refnum<vi>)
                n284 = call-by-ref "?"(reference=w376, "In"=w371, "Mode"=w375) -> ("Out"=w374:variant)  [unwired: 1 in, 2 out]
                n285 = Variant To Data(type=0.0, Variant=w374) -> (data=w372:dbl)  [unwired: 1 in, 1 out]
              }
            }
            n286 = local write "Value"(w366) -> ()
          }
          event "Save": Value Change {
            n287 = event-data() -> ("NewVal"=w377:bool)  [unwired: 1 in, 4 out]
            n288 = case shown="True" w377 {
              frame False {
              }
              frame True {
                n289 = flat-sequence {
                  frame #0 {
                    n290 = local read "Sequence File"() -> (w382:path)
                    n291 = local read "Chapter (us)"() -> (w380:string)
                    n292 = local read "Sequence"() -> (w379:string)
                    n293 = call "SaveSequenceString.vi"("Sequence"=w379, "Chapter"=w380) -> ("Sequence String"=w381:string)
                    n294 = call "CompileSequence.vi"("Sequence"=w379, "Chapter"=w380) -> ("Compiled Sequence"=w378:string)
                    n295 = Not Equal?(x=w382, y=path "") -> (x != y?=w384:bool)
                    n296 = case shown="True" w384 {
                      tunnel: w382 -> [_ w386]
                      tunnel: w381 -> [_ w385]
                      frame False {
                      }
                      frame True {
                        n297 = Write to Text File(file (use dialog)=w386, text=w385) -> ()  [unwired: 2 in, 3 out]
                      }
                    }
                    n298 = local write "CompiledSequence"(w378) -> ()
                  }
                  frame #1 {
                    n299 = local write "Save"(FALSE ("Compile")) -> ()
                    n300 = property on="Compile" class="Bool (strict)"("Val(Sgnl)"=TRUE ("Value (Signaling)")) -> ()  [unwired: 2 in, 2 out]
                  }
                }
              }
            }
          }
          event "Scan": Value Change {
            n301 = event-data() -> ("NewVal"=w389:bool)  [unwired: 1 in, 4 out]
            n302 = case shown="True" w389 {
              frame True {
                n303 = local read "Item"() -> (w391:string)
                n304 = Concatenate Strings(w391, "Scan-" ("string")) -> (w390:string)
                n305 = local read "Start"() -> (w400:dbl)
                n306 = flat-sequence {
                  tunnel: w390 -> [w418]
                  tunnel: w400 -> [w408]
                  tunnel: "Step" -> [w407]
                  tunnel: "End" -> [w413]
                  tunnel: w391 -> [w416]
                  tunnel: [w416] -> w398
                  tunnel: [w405] -> w397
                  tunnel: [w410] -> w396
                  tunnel: [w409] -> w395
                  tunnel: [w408] -> w394
                  tunnel: [w407] -> w393
                  tunnel: [w456] -> w399
                  tunnel: w398 -> [w456]
                  tunnel: w397 -> [w462]
                  tunnel: w396 -> [w461]
                  tunnel: w395 -> [w460]
                  tunnel: w394 -> [w459]
                  tunnel: w393 -> [w458]
                  tunnel: [w457] -> w392
                  tunnel: w399 -> [w501]
                  tunnel: w392 -> [w496]
                  frame #0 {
                    w422 = "\r\n"
                    n307 = Subtract(x=w413, y=w408) -> (x-y=w412:dbl)
                    n308 = property on="Average Counts or States" class="WFChart (strict)"("History Data"=dbl[] [], "XScale.Multiplier"=w407, "XScale.Offset"=w408, "XScale.Maximum"=w413) -> ()  [unwired: 2 in, 2 out]
                    n309 = local read "Parameter"() -> (w404:u16)
                    n310 = Divide(x=w412, y=w407) -> (x/y=w411:dbl)
                    n311 = case shown="Default" w416 {
                      tunnel: ["us" ("string") w445] -> w415
                      tunnel: [w436 w453] -> w414
                      tunnel: w404 -> [w432 w449]
                      frame "Time" {
                        n312 = local read "Durations"() -> (w443:dbl[])
                        n313 = local write "Durations Backup"(w443) -> ()
                        n314 = local read "Chapter (us)"() -> (w441:string)
                        n315 = local read "Sequence"() -> (w440:string)
                        n316 = call "SaveSequenceString.vi"("Sequence"=w440, "Chapter"=w441) -> ("Sequence String"=w438:string)
                        n317 = Number To Decimal String(number=w432) -> (decimal integer string=w434:string)  [unwired: 1 in]
                        n318 = Concatenate Strings("Sequence=\n{\n" ("string"), w438, "\n}\n" ("string"), "Index=" ("string"), w434, "\r\n") -> (w436:string)
                      }
                      frame Default {
                        w451 = u32 2 items=["Open", "Close", "Begin", "End", "Get", "Set"] ("Mode")
                        n319 = local read "Item Function"() -> (w450:refnum<vi>)
                        n320 = call-by-ref "?"(reference=w450, "In"=w449, "Mode"=w451) -> ("Out"=w448:variant)  [unwired: 1 in, 2 out]
                        n321 = Variant To Data(type=string[] [] ("Strings []"), Variant=w448) -> (data=w446:string[])  [unwired: 1 in, 1 out]
                        n322 = property on="Parameter" class="Ring (strict)"() -> ("RingText.Text"=w452:string)  [unwired: 2 in, 2 out]
                        n323 = Index Array(array=w446) -> (element #1=w445:string, element #2=w444:string)  [unwired: 2 in]
                        n324 = Concatenate Strings("Parameter=" ("string"), w452, "\r\n", w444) -> (w453:string)
                      }
                    }
                    n325 = Round Toward -Infinity(1:w411) -> (0:w406:dbl)
                    n326 = To Unsigned Long Integer(number=w406) -> (unsigned 32bit integer=w405:u32)
                    n327 = call <vilib>:"Space Constant.vi"() -> ("String"=w421:string)
                    n328 = Concatenate Strings(w421, w415) -> (w410:string)
                    n329 = Number To Fractional String(number=w408) -> (F-format string=w429:string)  [unwired: 3 in]
                    n330 = Number To Fractional String(number=w413) -> (F-format string=w427:string)  [unwired: 3 in]
                    n331 = Number To Fractional String(number=w407) -> (F-format string=w425:string)  [unwired: 3 in]
                    n332 = call "NewData.vi"("Prefix"=w418) -> ("data file name"=w419:string, "data file refnum"=w420:refnum<file>)  [unwired: 2 in]
                    n333 = local write "data file"(w419) -> ()
                    n334 = Concatenate Strings(w414, "Start=" ("string"), w429, w410, w422, "End=" ("string"), w427, w410, w422, "Step=" ("string"), w425, w410, w422, "Counts=" ("string"), w422, "{" ("string"), w422) -> (w430:string)
                    n335 = Write to Text File(file (use dialog)=w420, text=w430) -> (refnum out=w409:refnum<file>)  [unwired: 2 in, 2 out]
                  }
                  frame #1 {
                    n336 = while {
                      tunnel: w462 -> [w472]
                      tunnel: w461 -> [w468]
                      tunnel: w460 -> [w467]
                      shift-right: [w464] -> _
                      shift-left: w459 -> [w463]
                      tunnel: w458 -> [w466]
                      tunnel: [w465] -> w457
                      i -> [w473]
                      stop <- w469 continue-if-true
                      n337 = flat-sequence {
                        tunnel: w463 -> [w474]
                        tunnel: w468 -> [w483]
                        tunnel: w467 -> [w481]
                        tunnel: [w480] -> w465
                        tunnel: w463 -> [w479]
                        frame #0 {
                          n338 = local write "Value"(w474) -> ()
                        }
                        frame #1 {
                          n339 = property on="Set" class="Bool (strict)"("Val(Sgnl)"=TRUE ("Ready")) -> ()  [unwired: 2 in, 2 out]
                        }
                        frame #2 {
                          n340 = while {
                            stop <- w476 continue-if-true
                            n341 = local read "Set"() -> (w476:bool)
                          }
                        }
                        frame #3 {
                          n342 = property on="Data" class="Bool (strict)"("Val(Sgnl)"=TRUE ("Value (Signaling)")) -> ()  [unwired: 2 in, 2 out]
                        }
                        frame #4 {
                          n343 = while {
                            stop <- w478 continue-if-true
                            n344 = local read "Data"() -> (w478:bool)
                          }
                        }
                        frame #5 {
                          n345 = Number To Fractional String(number=w479) -> (F-format string=w489:string)  [unwired: 3 in]
                          n346 = local read "Counts"() -> (w484:u32[])
                          n347 = Concatenate Strings(w489, w483, "," ("string")) -> (w488:string)
                          n348 = for {
                            tunnel: w484 -> [w494] mode=indexing
                            shift-right: [w492] -> w485
                            shift-left: w488 -> [w491]
                            n349 = Number To Decimal String(number=w494) -> (decimal integer string=w493:string)  [unwired: 1 in]
                            n350 = call <vilib>:"Space Constant.vi"() -> ("String"=w490:string)
                            n351 = Concatenate Strings(w491, w490, w493) -> (w492:string)
                          }
                          n352 = Concatenate Strings(w485, "\r\n") -> (w486:string)
                          n353 = Write to Text File(file (use dialog)=w481, text=w486) -> (refnum out=w480:refnum<file>)  [unwired: 2 in, 2 out]
                        }
                      }
                      n354 = Add(x=w463, y=w466) -> (x+y=w464:dbl)
                      n355 = Less?(x=w473, y=w472) -> (x < y?=w471:bool)
                      n356 = local read "Scan"() -> (w470:bool)
                      n357 = And(x=w471, y=w470) -> (x .and. y?=w469:bool)
                    }
                  }
                  frame #2 {
                    n358 = case shown="\"Time\"" w501 {
                      frame "Time" {
                        n359 = local read "Durations Backup"() -> (w502:dbl[])
                        n360 = local write "Durations"(w502) -> ()
                      }
                      frame Default {
                        w505 = u32 3 items=["Open", "Close", "Begin", "End", "Get", "Set"] ("Mode")
                        n361 = local read "Item Function"() -> (w504:refnum<vi>)
                        n362 = local read "Parameter"() -> (w503:u16)
                        n363 = call-by-ref "?"(reference=w504, "In"=w503, "Mode"=w505) -> ()  [unwired: 1 in, 3 out]
                      }
                    }
                    n364 = local write "Scan"(FALSE ("Scan")) -> ()
                    n365 = Concatenate Strings("}" ("string"), "\r\n") -> (w497:string)
                    n366 = Write to Text File(file (use dialog)=w496, text=w497) -> (refnum out=w500:refnum<file>)  [unwired: 2 in, 2 out]
                    n367 = Close File(refnum=w500) -> ()  [unwired: 1 in, 2 out]
                  }
                }
              }
              frame False, Default {
              }
            }
          }
          event "Fit": Value Change {
            n368 = event-data() -> ("NewVal"=w506:bool)  [unwired: 1 in, 4 out]
            n369 = case shown="True" w506 {
              frame False {
              }
              frame True {
                n370 = local write "Fit"(FALSE ("Fit")) -> ()
                n371 = property on="Average Counts or States" class="WFChart (strict)"() -> ("History Data"=→"History":dbl[])  [unwired: 2 in, 2 out]
              }
            }
          }
          event "Clear": Value Change {
            n372 = event-data() -> ()  [unwired: 1 in, 6 out]
            n373 = property on="Average Counts or States" class="WFChart (strict)"("History Data"=dbl[] []) -> ()  [unwired: 2 in, 2 out]
          }
          event "Sequence File": Value Change {
            n374 = event-data() -> ("NewVal"=w511:path)  [unwired: 1 in, 4 out]
            n375 = call <vilib>:"Check if File or Folder Exists.vi"("path"=w511) -> ("file or folder exists?"=w512:bool, "dup path"=w510:path)  [unwired: 8 in, 1 out]
            n376 = case shown="True" w512 {
              tunnel: w510 -> [_ w513]
              frame False {
              }
              frame True {
                n377 = flat-sequence {
                  tunnel: w513 -> [w517]
                  frame #0 {
                    n378 = Read from Text File(file (use dialog)=w517) -> (text=w518:string)  [unwired: 3 in, 3 out]
                    n379 = call "LoadSequenceString.vi"("Sequence String"=w518) -> ("Chapter"=w516:string, "Sequence"=w515:string)
                    n380 = local write "Chapter (us)"(w516) -> ()
                    n381 = call "CompileSequence.vi"("Sequence"=w515, "Chapter"=w516) -> ("Compiled Sequence"=w514:string)
                    n382 = local write "Sequence"(w515) -> ()
                    n383 = local write "CompiledSequence"(w514) -> ()
                  }
                  frame #1 {
                    n384 = property on="Compile" class="Bool (strict)"("Val(Sgnl)"=TRUE ("Value (Signaling)")) -> ()  [unwired: 2 in, 2 out]
                  }
                }
              }
            }
          }
          event "Sweep": Value Change {
            n385 = event-data() -> ("NewVal"=w520:bool)  [unwired: 1 in, 4 out]
            n386 = case shown="True" w520 {
              frame False {
              }
              frame True {
                n387 = flat-sequence {
                  frame #0 {
                    n388 = local write "data file"("") -> ()
                    n389 = property on="Average Counts or States" class="WFChart (strict)"("History Data"=dbl[] []) -> (error out=w522:errorcluster)  [unwired: 2 in, 1 out]
                    n390 = property on="Average Counts or States" class="WFChart (strict)"(error in=w522, "XScale.Multiplier"=1.0 ("X Scale.Offset and Multiplier:Multiplier"), "XScale.Offset"=0.0 ("X Scale.Offset and Multiplier:Offset"), "XScale.Maximum"=100.0 ("X Scale.Range:Maximum")) -> ()  [unwired: 1 in, 2 out]
                  }
                  frame #1 {
                    n391 = while {
                      stop <- w527 continue-if-true
                      n392 = flat-sequence {
                        frame #0 {
                          n393 = property on="Data" class="Bool (strict)"("Val(Sgnl)"=TRUE ("Value (Signaling)")) -> ()  [unwired: 2 in, 2 out]
                        }
                        frame #1 {
                          n394 = while {
                            stop <- w529 continue-if-true
                            n395 = local read "Data"() -> (w529:bool)
                          }
                        }
                      }
                      n396 = local read "Sweep"() -> (w527:bool)
                    }
                  }
                }
              }
            }
          }
          event "Sequencer": Value Change {
            n397 = event-data() -> ("NewVal"=w530:bool)  [unwired: 1 in, 4 out]
          }
        }
      }
    }
    frame #3 {
      n398 = local read "Port"() -> (w531:refnum<visa-resource-name>)
      n399 = VISA Close(VISA resource name=w531) -> ()  [unwired: 1 in, 1 out]
    }
  }
